vi "Get One VR Crank Revolution Data.vi"(11 "Data In":dbl[](array[numeric])) -> (3 "One VR Crank Period":dbl[](array[numeric]), 5 "Selected Length":i32, 7 "Selected Offset":i32)   [LabVIEW 2019, in "Engine Simulation Toolkit System Explorer.lvlib"]
uses:
  Engine Simulation Toolkit System Explorer.lvlib
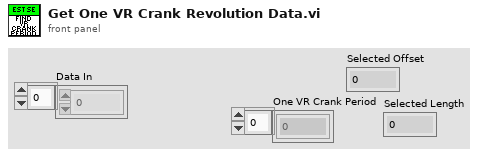
[diagram p1: front panel]
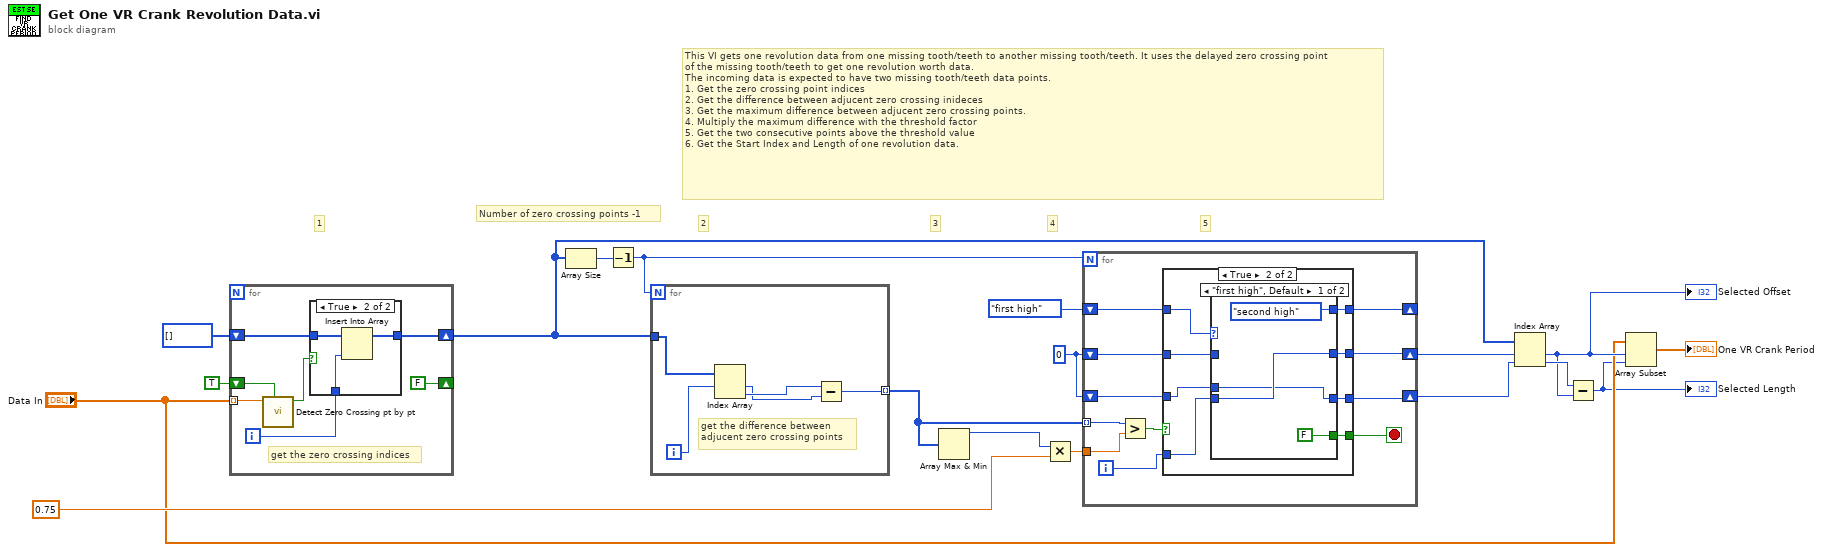
[diagram p0: block diagram]
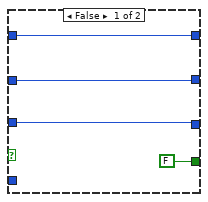
[diagram p2: hidden frame]
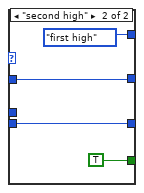
[diagram p3: hidden frame]
diagram:
  w18 = 0
  # "5"
  # "Number of zero crossing points -1"
  # "4"
  # "3"
  # "2"
  # "1"
  # "This VI gets one revolution data from one missing tooth/teeth to another missing tooth/teeth. It uses the delayed zero crossing point\nof the missing tooth/teeth to get one revolution worth data. \nThe incoming data is expected to have two missing tooth/teeth data points.\n1. Get the zero crossing point indices\n2. Get the difference between adjucent zero crossing inideces\n3. Get the maximum difference between adjucent zero crossing points.\n4. Multiply the maximum difference with the threshold factor\n5. Get the two consecutive points above the threshold value\n6. Get the Start Index and Length of one revolution data."
  n1 = for {
    tunnel: "Data In" -> [w25] mode=indexing
    shift-right: [w21] -> w8
    shift-left: i32[] [] -> [w23]
    shift-right: [FALSE] -> _
    shift-left: TRUE -> [w20]
    i -> [w22]
    # "get the zero crossing indices"
    n2 = call "Detect Zero Crossing pt by pt.vi"("initialize"=w20, "input data point"=w25) -> ("crossing"=w24:bool)  [unwired: 9 in]
    n3 = case shown="True" w24 {
      tunnel: w23 -> [w26 w29]
      tunnel: w22 -> [_ w28]
      tunnel: [w26 w27] -> w21
      frame False {
      }
      frame True {
        n4 = Insert Into Array(array=w29, new element=w28) -> (w27:i32[])  [unwired: 1 in]
      }
    }
  }
  n5 = Array Size(array=w8) -> (size(s)=w13:i32)
  n6 = Decrement(x=w13) -> (x-1=w6:i32)
  n7 = for {
    N: w6 -> [_]
    tunnel: w8 -> [w30]
    tunnel: [w31] -> w7 mode=indexing
    i -> [w34]
    # "get the difference between\nadjucent zero crossing points"
    n8 = Index Array(array=w30, index #1=w34) -> (element #1=w32:i32, element #2=w33:i32)  [unwired: 1 in]
    n9 = Subtract(x=w33, y=w32) -> (x-y=w31:i32)
  }
  n10 = Array Max & Min(array=w7) -> (max value=w14:i32)  [unwired: 3 out]
  n11 = Multiply(x=w14, y=sgl 0.75 ("Threshold Factor")) -> (x*y=w16:sgl)
  n12 = for {
    N: w6 -> [_]
    tunnel: w7 -> [w45] mode=indexing
    tunnel: w16 -> [w44]
    shift-right: [w39] -> _
    shift-left: enum16{"first high", "second high"}."first high" -> [w42]
    shift-right: [w40] -> w11
    shift-left: w18 -> [w37]
    shift-right: [w38] -> w10
    shift-left: w18 -> [w36]
    i -> [w41]
    stop <- w35 stop-if-true
    n13 = Greater?(x=w45, y=w44) -> (0:w43:bool)
    n14 = case shown="True" w43 {
      tunnel: w42 -> [w49 w57]
      tunnel: w41 -> [_ w56]
      tunnel: [w48 w55] -> w40
      tunnel: [w49 w54] -> w39
      tunnel: [w47 w53] -> w38
      tunnel: w37 -> [w48 w52]
      tunnel: w36 -> [w47 w51]
      tunnel: [FALSE w50] -> w35
      frame False {
      }
      frame True {
        n15 = case shown="\"first high\", Default" w57 {
          tunnel: w56 -> [w61 w65]
          tunnel: [w61 w64] -> w55
          tunnel: [enum16{"first high", "second high"}."second high" enum16{"first high", "second high"}."first high"] -> w54
          tunnel: [w59 w65] -> w53
          tunnel: w52 -> [_ w64]
          tunnel: w51 -> [w59 _]
          tunnel: [FALSE TRUE] -> w50
          frame "first high", Default {
          }
          frame "second high" {
          }
        }
      }
    }
  }
  n16 = Index Array(array=w8, index #1=w11, index #2=w10) -> (element #1=w5:i32, element #2=w9:i32)
  "Selected Offset" <- w5
  n17 = Subtract(x=w9, y=w5) -> (x-y=w2:i32)
  "Selected Length" <- w2
  n18 = Array Subset(array="Data In", index=w5, length=w2) -> (→"One VR Crank Period":dbl[])
